vi "Temp RT Target VI.vi"() -> ()   [LabVIEW 2018]
uses:
  <vilib>/Studica/Studica Toolkit/Background/DIO Channel.ctl
panel:
  in  "stop":bool
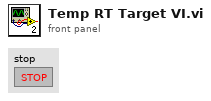
[diagram p1: front panel]
types:
  T1 = typedef "DIO Channel.ctl" = enum16{"Not Connected", "A/DIO1", "A/DIO2", "A/DIO3", "A/DIO4", "A/DIO5", "A/DIO6", "A/DIO7", "A/DIO13", "B/DIO1", "B/DIO2", "B/DIO3", "B/DIO4", "B/DIO5", "B/DIO6", "B/DIO7", "B/DIO13", "C/DIO0", "C/DIO1", "C/DIO2", "C/DIO3", "C/DIO4", "C/DIO5", "C/DIO6", "C/DIO7"}
  T2 = cluster{"DIO Channel":T1, "FPGA VI Reference Out":refnum<k20>}
  T3 = cluster{"xTargetSpeed":dbl, "yTargetSpeed":dbl, "wTargetSpeed":dbl}
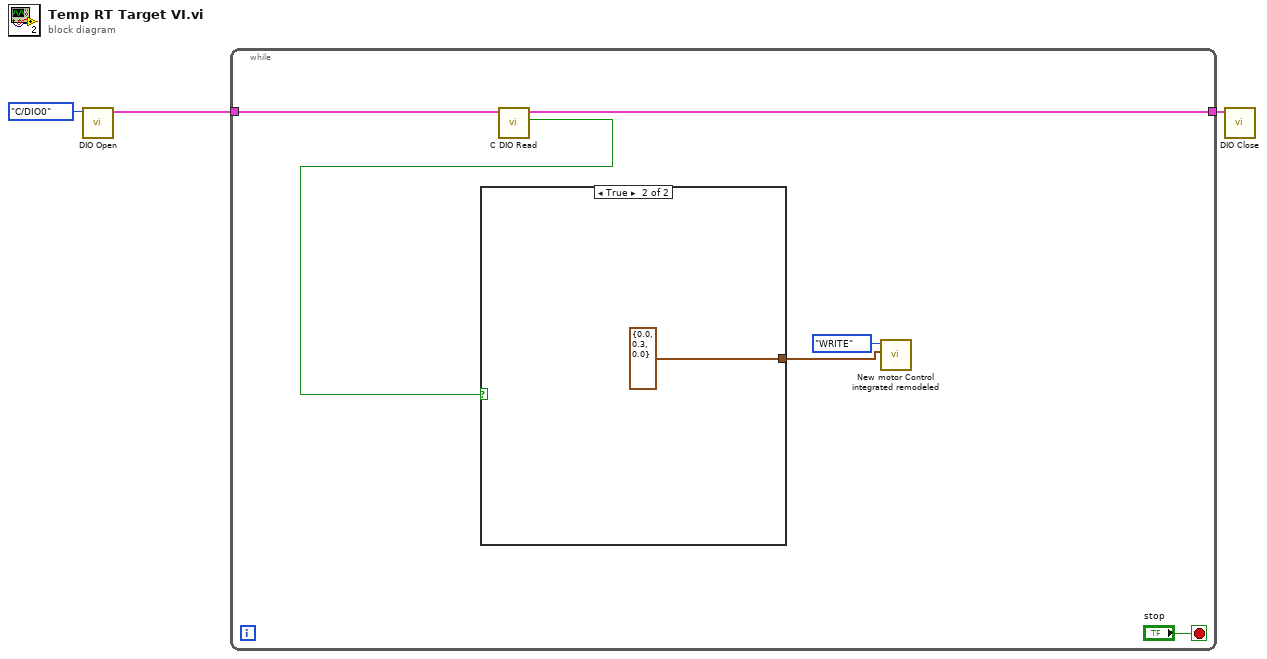
[diagram p0: block diagram]
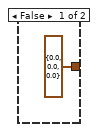
[diagram p2: hidden frame]
diagram:
  n1 = call <vilib>:"DIO Open.vi"("DIO Channel"=DIO_Channel."C/DIO0") -> ("DIO Info Out"=w3:T2)  [unwired: 9 in, 1 out]
  n2 = while {
    tunnel: w3 -> [w7]
    tunnel: [w6] -> w2
    stop <- "stop" stop-if-true
    n3 = call <vilib>:"C DIO Read.vi"("DIO Info In in"=w7) -> ("IN"=w5:bool, "DIO Info In out"=w6:T2)  [unwired: 8 in, 1 out]
    n4 = case shown="True" w5 {
      tunnel: [T3 {"xTargetSpeed"=0.0, "yTargetSpeed"=0.0, "wTargetSpeed"=0.0} ("Target Speed") T3 {"xTargetSpeed"=0.0, "yTargetSpeed"=0.3, "wTargetSpeed"=0.0} ("Target Speed")] -> w4
      frame False {
      }
      frame True {
      }
    }
    n5 = call "New motor Control integrated remodeled.vi"("States"=enum16{"RESET ENCODER", "WRITE", "READ", "INIT"}."WRITE", "Target Speed"=w4) -> ()  [unwired: 3 in, 2 out]
  }
  n6 = call <vilib>:"DIO Close.vi"("DIO Info In"=w2) -> ()  [unwired: 10 in, 1 out]
